vi "Error Query.vi"(0 "VISA resource name":refnum<visa-resource-name>, 11 "error in (no error)":errorcluster) -> (4 "VISA resource name out":refnum<visa-resource-name>, 8 "Error":i32, 10 "Error Message":string, 15 "error out":errorcluster)   [LabVIEW 2013, in "Yokogawa PZ4000.lvlib"]
doc: "This VI reads an error from the instrument. It expects to see errors in SCPI format (#,\"error message\")."
uses:
  Yokogawa PZ4000.lvlib
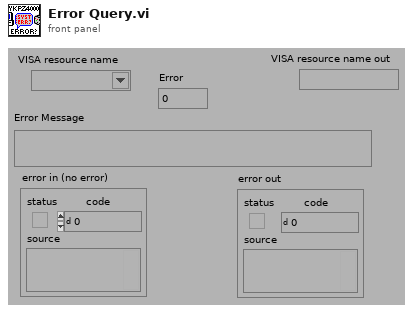
[diagram p1: front panel]
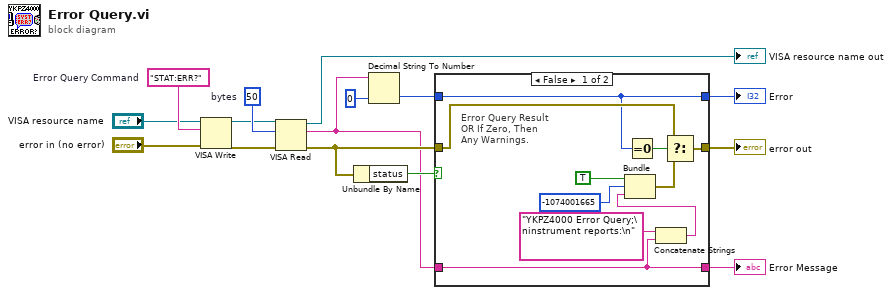
[diagram p0: block diagram]
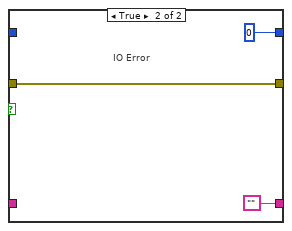
[diagram p2: hidden frame]
diagram:
  w10 = u32 50  # bytes
  w14 = "STAT:ERR?"  # Error Query Command
  n1 = VISA Write(VISA resource name="VISA resource name", write buffer=w14, error in (no error)="error in (no error)") -> (VISA resource name out=w9:refnum<visa-resource-name>, error out=w13:errorcluster)  [unwired: 1 out]
  n2 = VISA Read(VISA resource name=w9, byte count=w10, error in (no error)=w13) -> (VISA resource name out=→"VISA resource name out":refnum<visa-resource-name>, read buffer=w5:string, error out=w7:errorcluster)  [unwired: 1 out]
  n3 = Unbundle By Name(w7) -> ("status"=w6:bool)
  n4 = Decimal String To Number(string=w5, default (0L)=0) -> (number=w8:i32)  [unwired: 1 in, 1 out]
  n5 = case shown="False" w6 {
    tunnel: w5 -> [w23 _]
    tunnel: w7 -> [w19 w28]
    tunnel: [w20 w28] -> w3
    tunnel: [w23 ""] -> w2
    tunnel: [w16 0] -> w4
    tunnel: w8 -> [w16 _]
    frame False {
      # "Error Query Result\nOR If Zero, Then\nAny Warnings."
      n6 = Equal To 0?(x=w16) -> (x = 0?=w17:bool)
      n7 = Concatenate Strings("YKPZ4000 Error Query;\ninstrument reports:\n" ("Source"), w23) -> (w22:string)
      n8 = Bundle("Status"=TRUE, "Code"=-1074001665, w22) -> (w21:cluster{"Status":bool, "Code":i32, string})  [unwired: 1 in]
      n9 = Select(t=w19, s=w17, f=w21) -> (s? t:f=w20:errorcluster)
    }
    frame True {
      # "IO Error"
    }
  }
  "Error Message" <- w2
  "error out" <- w3
  "Error" <- w4
